vi "ProgramRemote.vi"(0 "Universal Robot.lvclass in":refnum<class "Universal Robot.lvclass">, 3 "Remote":T1, 5 "error in (no error)":errorcluster) -> (14 "Universal Robot.lvclass out":refnum<class "Universal Robot.lvclass">, 19 "error out":errorcluster)   [LabVIEW 2016, in "Universal Robot.lvclass"]
uses:
  Universal Robot.lvclass
  ProgramControlEvent.ctl
  Universal Robot.lvclass/Universal Robot.ctl
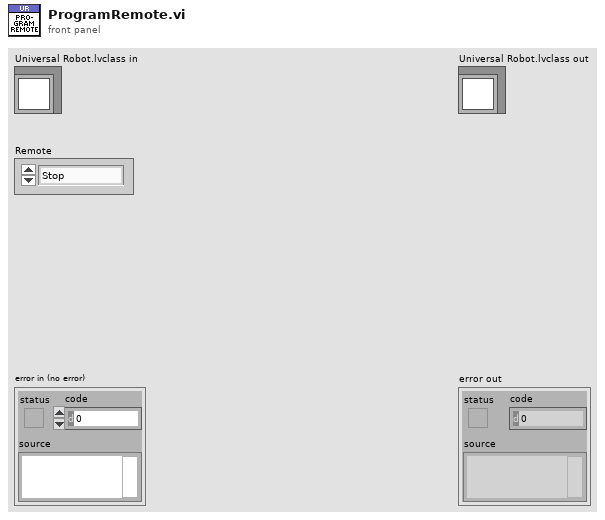
[diagram p1: front panel]
types:
  T1 = typedef "Universal Robot.lvclass/ProgramControlEvent.ctl" = enum16{"Stop", "Pause"}
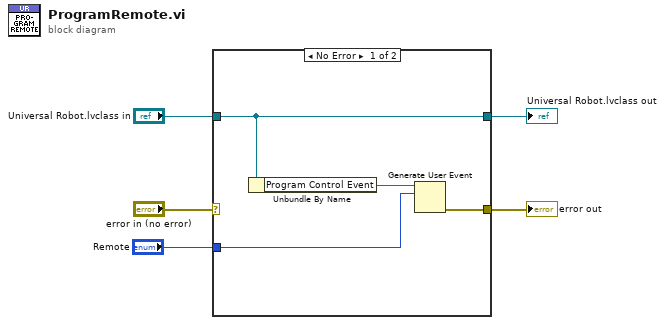
[diagram p0: block diagram]
diagram:
  n1 = case shown="No Error" "error in (no error)" {
    selector: "error in (no error)" -> [_ w11]
    tunnel: [w6 w11] -> w4
    tunnel: "Universal Robot.lvclass in" -> [w9 w10]
    tunnel: [w9 w10] -> w2
    tunnel: "Remote" -> [w7 _]
    frame No Error {
      n2 = Unbundle By Name(w9) -> ("Program Control Event"=w8:refnum<user-event>)
      n3 = Generate User Event(user event=w8, event data cluster=w7) -> (error out=w6:errorcluster)  [unwired: 2 in, 1 out]
    }
    frame Error {
    }
  }
  "error out" <- w4
  "Universal Robot.lvclass out" <- w2
